vi "Drive Controller.vi"(8 "error in":errorcluster) -> ()   [LabVIEW 2019]
doc: "This VI executes continuously carrying out the current operation and responding to updates or new operation requests. It will often contain the timing or control code that is difficult to place directly in TeleOp. This VI generally opens all sensors and motors and isolates the rest of the robot code from knowing implementation details of how the operations are carried out."
uses:
  <vilib>/Rock Robotics/WPI/Framework/Completion Status.ctl
  Drive Setpoints.ctl
  Drive Operations.ctl
  <vilib>/Rock Robotics/WPI/SafetyOutput/WPI_SafetyOutputConfigMenu.ctl
  <vilib>/Rock Robotics/SystemInterfaces/DIO/FPGA_DIOChannel.ctl
  <vilib>/Rock Robotics/WPI/Solenoid/WPI_SolenoidChannel.ctl
  <vilib>/Rock Robotics/WPI/Solenoid/WPI_SolenoidValue.ctl
  <vilib>/Rock Robotics/WPI/Counter/WPI_CounterDigitalInputToDigitalSource.vi
  <vilib>/Rock Robotics/WPI/Solenoid/WPI_SolenoidOpenDouble.vi
  <vilib>/Rock Robotics/WPI/Solenoid/WPI_SolenoidSetEnum.vi
  <vilib>/Rock Robotics/WPI/RobotDrive/WPI_RobotDriveOpen4MotorWithExistingMotors.vi
  Drive Globals.vi
  <vilib>/Rock Robotics/WPI/RobotDrive/WPI_RobotDriveOpen2MotorWithVictorSPX.vi
panel:
  out "Right Drive Velocity":dbl
  out "Left Drive Velocity":dbl
  in  "Interactive Values":T1
  in  "Buttons":cluster{"Execute Cmd":bool, "Abort Cmd":bool}
  out "Command Timing":cluster{"Start Time (ms)":u32, "Iterations":i32}
  out "Status":T3
  out "Setpoints":T4(graph)
  out "Current\nCmd":string
  # "Tip: The graph shows the motor setpoints. It may also be helpful to observe inputs and sensor values.\nYou may also want to display tuning or debugging controls."
  # "Interactive Command: You may fill in the settings for a command\nand schedule it with the Execute button. You can observe and abort\nany command while fine tuning the code for the controller."
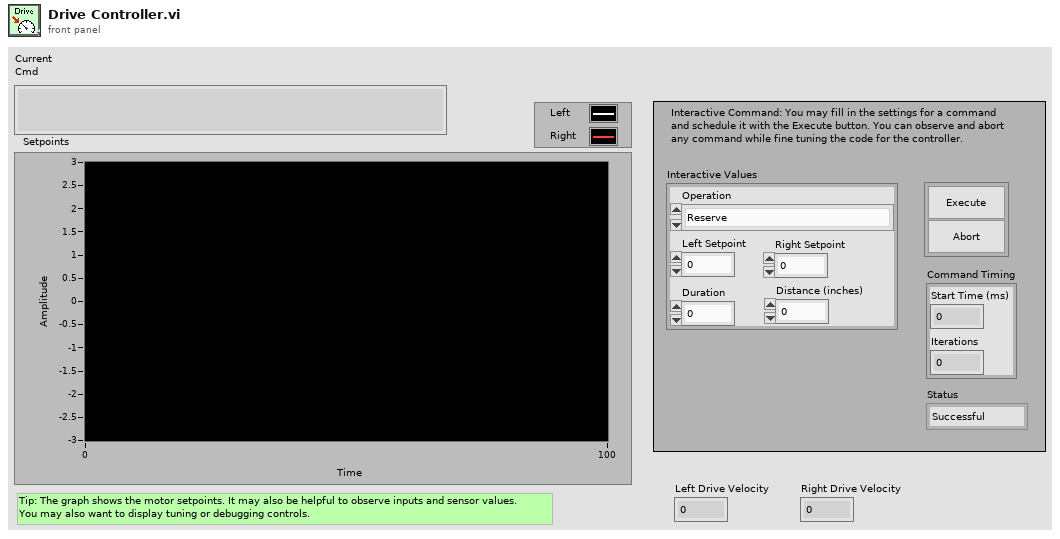
[diagram p1: front panel]
types:
  T1 = typedef "Drive Setpoints.ctl" = cluster{"Operation":T2, "Left Setpoint":dbl, "Right Setpoint":dbl, "Duration":dbl, "Distance (inches)":dbl}
  T2 = typedef "Drive Operations.ctl" = enum16{"Reserve", "Read Current", "Immediate", "Drive for Time", "Drive for Distance"}
  T3 = typedef "Completion Status.ctl" = enum16{"Successful", "Aborted", "Incomplete"}
  T4 = cluster{"Left Setpoint":dbl, "Right Setpoint":dbl}
  T5 = typedef "WPI_SolenoidValue.ctl" = enum16{"Off", "On", "Forward", "Reverse"}
  T6 = typedef "WPI_SolenoidChannel.ctl" = enum8{"Solenoid 0", "Solenoid 1", "Solenoid 2", "Solenoid 3", "Solenoid 4", "Solenoid 5", "Solenoid 6", "Solenoid 7", "Invalid"}
  T7 = typedef "FPGA_DIOChannel.ctl" = enum8{"DIO 0", "DIO 1", "DIO 2", "DIO 3", "DIO 4", "DIO 5", "DIO 6", "DIO 7", "DIO 8", "DIO 9", "DIO MXP 0", "DIO MXP 1", "DIO MXP 2", "DIO MXP 3", "DIO MXP 4", "DIO MXP 5", "DIO MXP 6", "DIO MXP 7", "DIO MXP 8", "DIO MXP 9", "DIO MXP 10", "DIO MXP 11", "DIO MXP 12", "DIO MXP 13", "DIO MXP 14", "DIO MXP 15", "SPI Port CS1", "SPI Port CS2", "SPI Port CS3", "SPI Port MISO", "SPI Port MOSI", "Invalid"}
  T8 = typedef "WPI_SafetyOutputConfigMenu.ctl" = enum16{"Enable", "Disable"}
  T9 = typedef "WPI_MotorControlDeviceRef.ctl" = cluster{"DeviceStatus":errorcluster, "Type":T10, "PWM":cluster{"PWM Channel":T11, "DeadBand":T12}, "CAN":cluster{"Device Number":u8, "SetOutput VI Ref":variant, "GetOutput VI Ref":variant, "Enable VI Ref":variant, "Disable VI Ref":variant, "Data":variant}, "Invert":bool, "DIO PWM":cluster{"PWM \"Enable\" Channel":T11, "DIOChannel":T7, "PWM Rate":dbl}}
  T10 = typedef "WPI_MotorControlType.ctl" = enum16{"PWM", "CAN", "DIO PWM"}
  T11 = typedef "FPGA_DIOPWMChannel.ctl" = enum8{"PWM 0", "PWM 1", "PWM 2", "PWM 3", "PWM 4", "PWM 5", "PWM 6", "PWM 7", "PWM 8", "PWM 9", "PWM MXP 0", "PWM MXP 1", "PWM MXP 2", "PWM MXP 3", "PWM MXP 4", "PWM MXP 5", "PWM MXP 6", "PWM MXP 7", "PWM MXP 8", "PWM MXP 9", "Invalid"}
  T12 = typedef "WPI_PWMDeadband.ctl" = cluster{"Name":string, "maxPositivePwm":i32, "minPositivePwm":i32, "centerPwm":i32, "maxNegativePwm":i32, "minNegativePwm":i32, "angularRange":u16}
  T13 = typedef "WPI_DigitalInputDevRef.ctl" = cluster{"DevStatus":errorcluster, "DIO Channel":T7}
  T14 = typedef "FPGA_CounterEncoderSourceConvertionLVSourceType.ctl" = cluster{"DevStatus":errorcluster, "AnalogTriggerMode?":bool, "DigitalMode":cluster{"DIO Channel":T15}, "AnalogTriggerMode":cluster{"AnalogTriggerIndex":T16, "OutputType":T17}}
  T15 = typedef "FPGA_DIODigitalSourceChannel.ctl" = enum8{"DIO 0", "DIO 1", "DIO 2", "DIO 3", "DIO 4", "DIO 5", "DIO 6", "DIO 7", "DIO 8", "DIO 9", "DIO MXP 0", "DIO MXP 1", "DIO MXP 2", "DIO MXP 3", "DIO MXP 4", "DIO MXP 5", "DIO MXP 6", "DIO MXP 7", "DIO MXP 8", "DIO MXP 9", "DIO MXP 10", "DIO MXP 11", "DIO MXP 12", "DIO MXP 13", "DIO MXP 14", "DIO MXP 15", "SPI Port CS1", "SPI Port CS2", "SPI Port CS3", "SPI Port MISO", "SPI Port MOSI", "Disabled"}
  T16 = typedef "FPGA_AnalogTriggerIndex.ctl" = enum8{"Trig 0", "Trig 1", "Trig 2", "Trig 3", "Trig 4", "Trig 5", "Trig 6", "Trig 7", "Invalid"}
  T17 = typedef "FPGA_AnalogTriggerOutType.ctl" = enum16{"InWindow", "TriggerState", "Rising", "Falling"}
  T18 = typedef "WPI_RobotDriveDevRef.ctl" = cluster{"DevStatus":errorcluster, "Motors[]":T9[], "Square Inputs":bool, "Max Output":dbl}
  T19 = typedef "WPI_SolenoidDevRef.ctl" = cluster{"DevStatus":errorcluster, "Pneumatics Control Module":u8, "Forward Solenoid Channel":T6, "Reverse Solenoid Channel":T6}
  T20 = typedef "WPI_EncoderDevRef.ctl" = cluster{"DevStatus":errorcluster, "EncoderIndex":T21, "CounterIndex":T22, "DistancePerCount":dbl, "Decoding Type":T23}
  T21 = typedef "FPGA_EncoderIdx.ctl" = enum8{"Enc 0", "Enc 1", "Enc 2", "Enc 3", "Enc 4", "Enc 5", "Enc 6", "Enc 7", "Invalid"}
  T22 = typedef "FPGA_CounterCtrSystemIndex.ctl" = enum8{"Ctr 0", "Ctr 1", "Ctr 2", "Ctr 3", "Ctr 4", "Ctr 5", "Ctr 6", "Ctr 7", "Invalid"}
  T23 = typedef "WPI_EncoderType.ctl" = enum16{"1x", "2x", "4x"}
  T24 = typedef "Command Status Info.ctl" = cluster{"Name":string, "Status":T3, "notifier out":T25}
  T25 = typedef "Completion Notifier.ctl" = refnum<notifier>
  T26 = cluster{"SubSystem Data":T1, cluster{"Start Time (ms)":u32, "Iterations":i32}, cluster{"Command Info":T24, "Description":string, "Default Command":T1, "queue out":refnum<queue>, "Subsystem Name":string}}
  T27 = cluster{"SubSystem Data":T1, cluster{"Start Time (ms)":u32, "Iterations":i32}, "Default Command Arguments":cluster{"Command Info":T24, "Description":string, "Default Command":T1, "queue out":refnum<queue>, "Subsystem Name":string}}
  T28 = cluster{"Sensor Velocity":dbl, "Sensor Velocity":dbl}
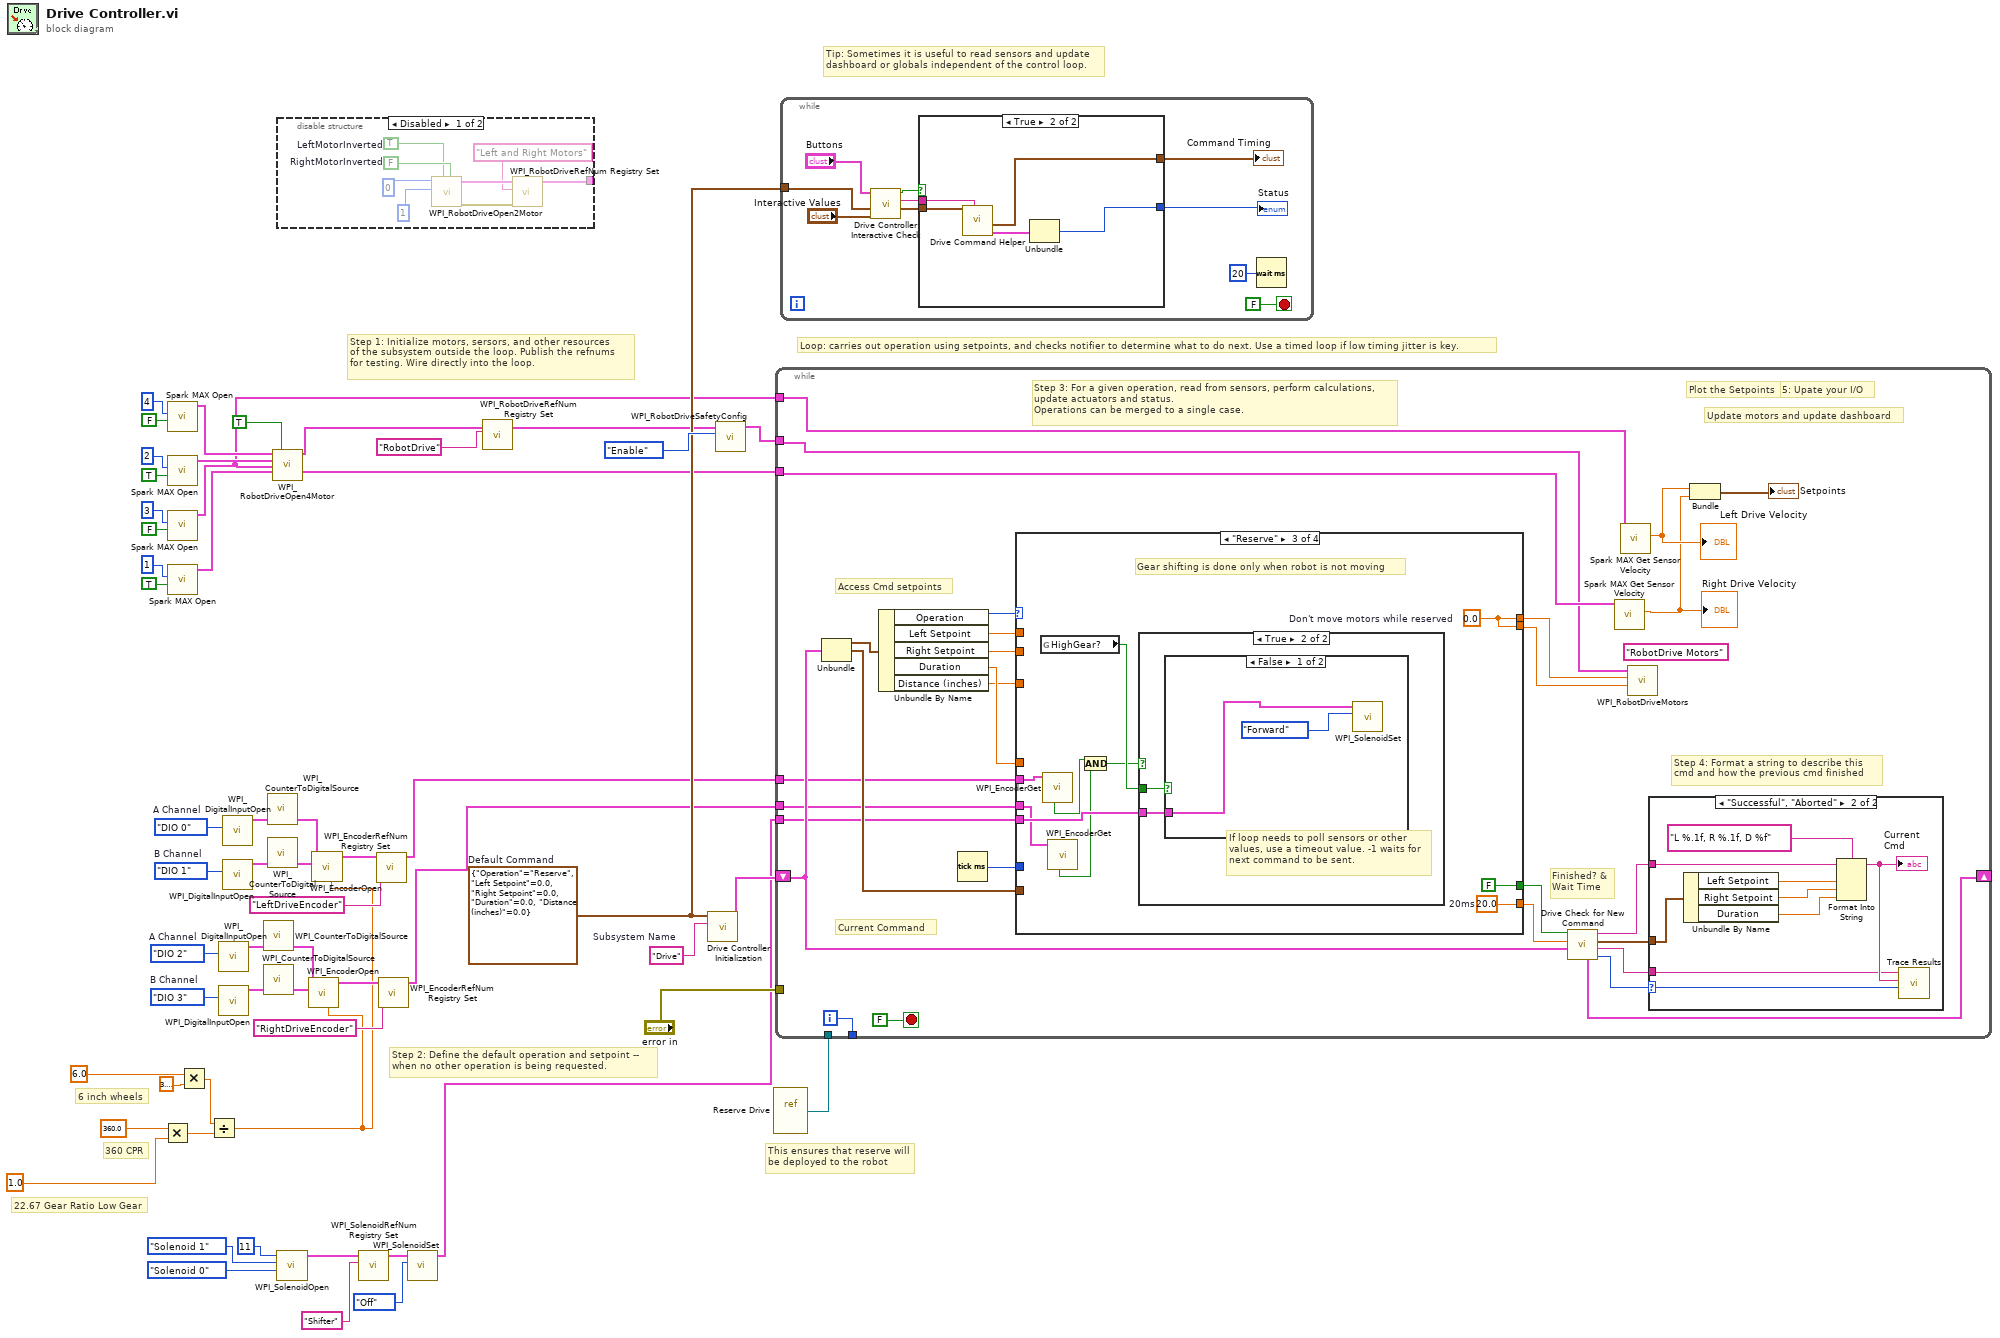
[diagram p0: block diagram]
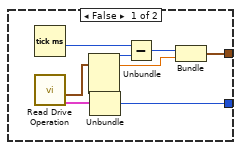
[diagram p3: hidden frame]
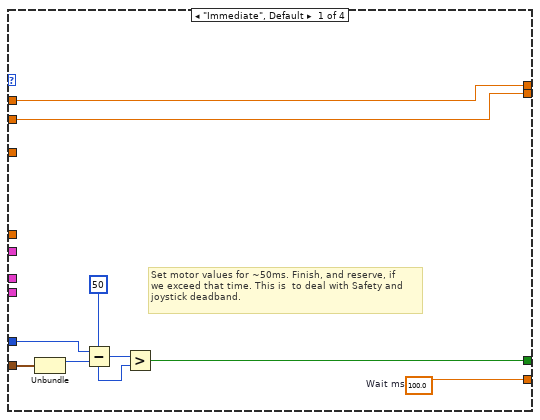
[diagram p5: hidden frame]
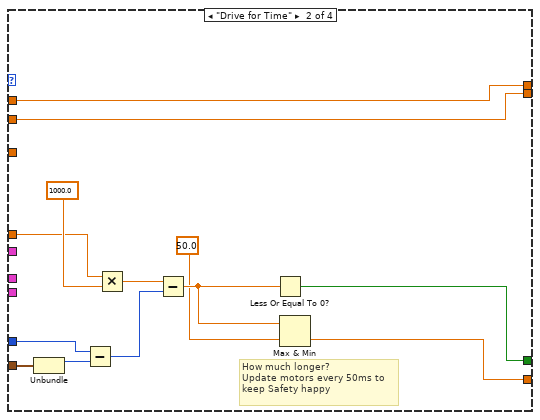
[diagram p6: hidden frame]
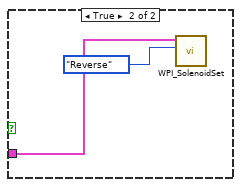
[diagram p8: hidden frame]
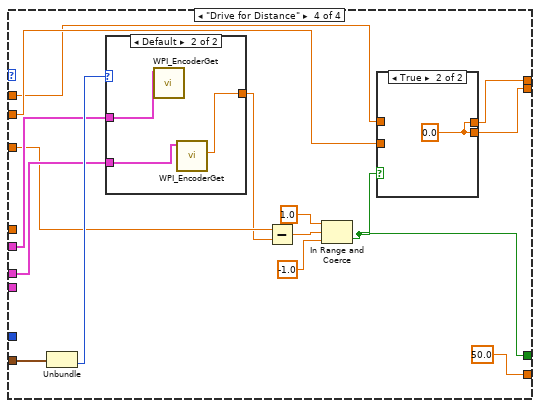
[diagram p9: hidden frame]
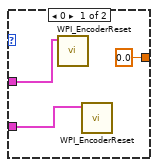
[diagram p11: hidden frame]
diagram:
  w33 = FPGA_DIOChannel."DIO 3"  # B Channel
  w32 = FPGA_DIOChannel."DIO 2"  # A Channel
  w39 = FPGA_DIOChannel."DIO 1"  # B Channel
  w38 = FPGA_DIOChannel."DIO 0"  # A Channel
  w50 = T1 {"Operation"=enum."Reserve", "Left Setpoint"=0.0, "Right Setpoint"=0.0, "Duration"=0.0, "Distance (inches)"=0.0}  # Default Command
  w56 = "Drive"  # Subsystem Name
  # "6 inch wheels"
  # "22.67 Gear Ratio Low Gear"
  # "360 CPR"
  # "This ensures that reserve will\nbe deployed to the robot"
  # "Tip: Sometimes it is useful to read sensors and update\ndashboard or globals independent of the control loop."
  # "Step 2: Define the default operation and setpoint --\nwhen no other operation is being requested."
  # "Step 1: Initialize motors, sersors, and other resources\nof the subsystem outside the loop. Publish the refnums\nfor testing. Wire directly into the loop."
  # "Loop: carries out operation using setpoints, and checks notifier to determine what to do next. Use a timed loop if low timing jitter is key."
  n1 = Multiply(x=360.0, y=1.0) -> (x*y=w4:dbl)
  n2 = call <vilib>:"Spark MAX Open.vi"("Invert"=FALSE, "Device Number"=u8 4) -> ("MotorControlDeviceRef"=w40:T9)  [unwired: 8 in, 1 out]
  n3 = call <vilib>:"Spark MAX Open.vi"("Invert"=TRUE, "Device Number"=u8 2) -> ("MotorControlDeviceRef"=w41:T9)  [unwired: 8 in, 1 out]
  n4 = call <vilib>:"Spark MAX Open.vi"("Invert"=FALSE, "Device Number"=u8 3) -> ("MotorControlDeviceRef"=w2:T9)  [unwired: 8 in, 1 out]
  n5 = call <vilib>:"Spark MAX Open.vi"("Invert"=TRUE, "Device Number"=u8 1) -> ("MotorControlDeviceRef"=w1:T9)  [unwired: 8 in, 1 out]
  n6 = Multiply(x=6.0 ("DistancePerCount"), y=3.141592653589793) -> (x*y=w5:dbl)
  n7 = Divide(x=w5, y=w4) -> (x/y=w3:dbl)
  n8 = call <vilib>:"WPI_DigitalInputOpen.vi"("DIO Channel"=w32) -> ("DigitalInputDevRef"=w29:T13)  [unwired: 1 in, 9 out]
  n9 = call <vilib>:"WPI_DigitalInputOpen.vi"("DIO Channel"=w33) -> ("DigitalInputDevRef"=w30:T13)  [unwired: 1 in, 9 out]
  n10 = call <vilib>:"WPI_DigitalInputOpen.vi"("DIO Channel"=w38) -> ("DigitalInputDevRef"=w35:T13)  [unwired: 1 in, 9 out]
  n11 = call <vilib>:"WPI_DigitalInputOpen.vi"("DIO Channel"=w39) -> ("DigitalInputDevRef"=w36:T13)  [unwired: 1 in, 9 out]
  n12 = call-poly <vilib>:"WPI_CounterToDigitalSource.vi"("DigitalInputDevRef"=w29) -> ("Digital Source"=w28:T14)  [unwired: 6 out]
  n13 = call-poly <vilib>:"WPI_CounterToDigitalSource.vi"("DigitalInputDevRef"=w30) -> ("Digital Source"=w31:T14)  [unwired: 6 out]
  n14 = call-poly <vilib>:"WPI_CounterToDigitalSource.vi"("DigitalInputDevRef"=w35) -> ("Digital Source"=w34:T14)  [unwired: 6 out]
  n15 = call-poly <vilib>:"WPI_CounterToDigitalSource.vi"("DigitalInputDevRef"=w36) -> ("Digital Source"=w37:T14)  [unwired: 6 out]
  n16 = call-poly <vilib>:"WPI_RobotDriveOpen4Motor.vi"("Rear Left Motor Dev Ref"=w40, "Square Inputs"=TRUE, "Rear Right Motor Dev Ref"=w41, "Front Left Motor Dev Ref"=w2, "Front Right Motor Dev Ref"=w1) -> ("RobotDriveDevRef"=w43:T18)  [unwired: 9 in, 1 out]
  n17 = call-poly <vilib>:"WPI_SolenoidOpen.vi"("Reverse Solenoid Channel"=WPI_SolenoidChannel."Solenoid 0", "Forward Solenoid Channel"=WPI_SolenoidChannel."Solenoid 1", "Pneumatics Control Module (0)"=11) -> ("SolenoidDevRef"=w19:T19)  [unwired: 7 in, 1 out]
  n18 = disable-structure shown="Disabled" {
    disable-tunnel: [w57 _] -> _
    frame Disabled {
      w61 = TRUE  # LeftMotorInverted
      w62 = FALSE  # RightMotorInverted
      n19 = call-poly <vilib>:"WPI_RobotDriveOpen2Motor.vi"("Right Motor Inverted"=w62, "Left Motor Inverted"=w61, "Right Motor"=u8 1 ("Left Motor"), "Left Motor"=u8 0) -> ("error out"=w58:errorcluster, "RobotDriveDevRef"=w60:T18)  [unwired: 1 in, 5 out]
      n20 = call <vilib>:"WPI_RobotDriveRefNum Registry Set.vi"("error in (no error)"=w58, "refnum name"="Left and Right Motors", "RobotDriveDevRef"=w60) -> ("RobotDriveDevRef"=w57:T18)  [unwired: 1 in, 7 out]
    }
    frame Enabled {
    }
  }
  n21 = call <vilib>:"WPI_EncoderOpen.vi"("DistancePerCount"=w3, "BSource"=w31, "ASource"=w28) -> ("EncoderDevRef"=w25:T20)  [unwired: 5 in, 3 out]
  n22 = call <vilib>:"WPI_EncoderOpen.vi"("DistancePerCount"=w3, "BSource"=w37, "ASource"=w34) -> ("EncoderDevRef"=w27:T20)  [unwired: 5 in, 3 out]
  n23 = call <vilib>:"WPI_SolenoidRefNum Registry Set.vi"("refnum name"="Shifter", "SolenoidDevRef"=w19) -> ("SolenoidDevRef"=w18:T19)  [unwired: 8 in, 1 out]
  n24 = call <vilib>:"WPI_EncoderRefNum Registry Set.vi"("refnum name"="LeftDriveEncoder", "EncoderDevRef"=w27) -> ("EncoderDevRef"=w23:T20)  [unwired: 8 in, 1 out]
  n25 = call <vilib>:"WPI_EncoderRefNum Registry Set.vi"("refnum name"="RightDriveEncoder", "EncoderDevRef"=w25) -> ("EncoderDevRef"=w14:T20)  [unwired: 8 in, 1 out]
  n26 = call-poly <vilib>:"WPI_SolenoidSet.vi"("Value"=WPI_SolenoidValue."Off", "SolenoidDevRef"=w18) -> ("SolenoidDevRef"=w15:T19)  [unwired: 8 in, 1 out]
  n27 = call <vilib>:"WPI_RobotDriveRefNum Registry Set.vi"("refnum name"="RobotDrive", "RobotDriveDevRef"=w43) -> ("RobotDriveDevRef"=w44:T18)  [unwired: 2 in, 7 out]
  n28 = call "Drive Controller Initialization.vi"("Subsystem Name"=w56, "Default Command"=w50) -> ("Current Command"=w52:T26)  [unwired: 9 in]
  n29 = call <vilib>:"WPI_RobotDriveSafetyConfig.vi"("mode"=WPI_SafetyOutputConfigMenu."Enable", "RobotDriveDevRef"=w44) -> ("RobotDriveDevRef"=w54:T18)  [unwired: 8 in, 1 out]
  n30 = vi-ref "Reserve Drive.vi"() -> (w51:refnum<vi>)
  n31 = while {
    shift-right: [w81] -> _
    shift-left: w52 -> [w74]
    tunnel: [w92] -> _
    tunnel: w54 -> [w66]
    tunnel: "error in" -> [_]
    tunnel: w51 -> [_]
    tunnel: w23 -> [w73]
    tunnel: w15 -> [w72]
    tunnel: w14 -> [w71]
    tunnel: w2 -> [w69]
    tunnel: w1 -> [w68]
    i -> [w92]
    stop <- FALSE stop-if-true
    (unwired) "RobotDrive Motors" ("Name")
    # "Step 5: Upate your I/O"
    # "Step 4: Format a string to describe this\ncmd and how the previous cmd finished"
    # "Current Command"
    # "Update motors and update dashboard"
    # "Plot the Setpoints"
    # "Access Cmd setpoints"
    # "Finished? &\nWait Time"
    # "Step 3: For a given operation, read from sensors, perform calculations,\nupdate actuators and status.\nOperations can be merged to a single case."
    n32 = Unbundle(w74) -> ("SubSystem Data"=w88:T1, w75:cluster{"Start Time (ms)":u32, "Iterations":i32})  [unwired: 1 out]
    n33 = Unbundle By Name(w88) -> ("Operation"=w87:T2, "Left Setpoint"=w86:dbl, "Right Setpoint"=w85:dbl, "Duration"=w84:dbl, "Distance (inches)"=w70:dbl)
    n34 = Tick Count (ms)() -> (millisecond timer value=w83:u32)
    n35 = case shown="\"Reserve\"" w87 {
      tunnel: [w111 w112 w134 50.0 ("20ms")] -> w80
      tunnel: [w104 w119 FALSE ("ignore previous (F)") w144] -> w79
      tunnel: w75 -> [w103 w121 _ w155]
      tunnel: [w110 w118 w132 w148] -> w90
      tunnel: [w109 w117 w132 w149] -> w89
      tunnel: w86 -> [w110 w118 _ w150]
      tunnel: w85 -> [w109 w117 _ w151]
      tunnel: w84 -> [_ w116 _ _]
      tunnel: w83 -> [w105 w115 _ _]
      tunnel: w73 -> [_ _ w131 w153]
      tunnel: w72 -> [_ _ w130 _]
      tunnel: w71 -> [_ _ w127 w152]
      tunnel: w70 -> [_ _ _ w146]
      frame "Immediate", Default {
        w111 = 100.0  # Wait ms
        # "Set motor values for ~50ms. Finish, and reserve, if\nwe exceed that time. This is  to deal with Safety and\njoystick deadband."
        n36 = Unbundle(w103) -> ("Start Time (ms)"=w106:u32)  [unwired: 1 out]
        n37 = Subtract(x=w105, y=w106) -> (x-y=w107:u32)
        n38 = Greater?(x=w107, y=u8 50 ("Left Motor")) -> (0:w104:bool)
      }
      frame "Drive for Time" {
        # "How much longer?\nUpdate motors every 50ms to\nkeep Safety happy"
        n39 = Unbundle(w121) -> ("Start Time (ms)"=w120:u32)  [unwired: 1 out]
        n40 = Subtract(x=w115, y=w120) -> (x-y=w124:u32)
        n41 = Multiply(x=w116, y=1000.0) -> (x*y=w123:dbl)
        n42 = Subtract(x=w123, y=w124) -> (x-y=w114:dbl)
        n43 = Less Or Equal To 0?(x=w114) -> (x <= 0?=w119:bool)
        n44 = Max & Min(x=w114, y=50.0) -> (min(x,y)=w112:dbl)  [unwired: 1 out]
      }
      frame "Reserve" {
        w132 = 0.0  # Don't move motors while reserved
        w134 = 20.0  # 20ms
        # "Gear shifting is done only when robot is not moving"
        n45 = global read "Drive Globals.vi" "HighGear?"() -> (w129:bool)
        n46 = call <vilib>:"WPI_EncoderGet.vi"("EncoderDevRef"=w131) -> ("Stopped"=w128:bool)  [unwired: 5 in, 5 out]
        n47 = call <vilib>:"WPI_EncoderGet.vi"("EncoderDevRef"=w127) -> ("Stopped"=w126:bool)  [unwired: 5 in, 5 out]
        n48 = And(x=w128, y=w126) -> (x .and. y?=w125:bool)
        n49 = case shown="True" w125 {
          tunnel: w130 -> [_ w136]
          tunnel: w129 -> [_ w135]
          frame False {
          }
          frame True {
            # "If loop needs to poll sensors or other\nvalues, use a timeout value. -1 waits for\nnext command to be sent."
            n50 = case shown="False" w135 {
              tunnel: w136 -> [w137 w140]
              frame False {
                n51 = call-poly <vilib>:"WPI_SolenoidSet.vi"("Value"=WPI_SolenoidValue."Forward", "SolenoidDevRef"=w137) -> ()  [unwired: 8 in, 2 out]
              }
              frame True {
                n52 = call-poly <vilib>:"WPI_SolenoidSet.vi"("Value"=WPI_SolenoidValue."Reverse", "SolenoidDevRef"=w140) -> ()  [unwired: 8 in, 2 out]
              }
            }
          }
        }
      }
      frame "Drive for Distance" {
        n53 = Unbundle(w155) -> ("Iterations"=w154:i32)  [unwired: 1 out]
        n54 = case shown="Default" w154 {
          tunnel: w153 -> [w161 w164]
          tunnel: w152 -> [w160 w163]
          tunnel: [0.0 ("Distance") w162] -> w145
          frame 0 {
            n55 = call <vilib>:"WPI_EncoderReset.vi"("EncoderDevRef"=w161) -> ()  [unwired: 9 in, 2 out]
            n56 = call <vilib>:"WPI_EncoderReset.vi"("EncoderDevRef"=w160) -> ()  [unwired: 9 in, 2 out]
          }
          frame Default {
            n57 = call <vilib>:"WPI_EncoderGet.vi"("EncoderDevRef"=w164) -> ()  [unwired: 5 in, 6 out]
            n58 = call <vilib>:"WPI_EncoderGet.vi"("EncoderDevRef"=w163) -> ("Distance"=w162:dbl)  [unwired: 5 in, 5 out]
          }
        }
        n59 = Subtract(x=w146, y=w145) -> (x-y=w143:dbl)
        n60 = In Range and Coerce(upper limit=1.0, x=w143, lower limit=-1.0) -> (In Range?=w144:bool)  [unwired: 1 out]
        n61 = case shown="True" w144 {
          tunnel: w151 -> [w156 _]
          tunnel: w150 -> [w157 _]
          tunnel: [w156 w158] -> w149
          tunnel: [w157 w158] -> w148
          frame False {
          }
          frame True {
            w158 = 0.0
          }
        }
      }
    }
    n62 = call "Drive Check for New Command.vi"("input cluster"=w74, "Wait time (ms)"=w80, "Finished?"=w79) -> ("Completion"=w82:T3, "Subsystem Name"=w76:string, "Current Command"=w77:T1, "Initial Trace String"=w78:string, "Next Command"=w81:T27)  [unwired: 4 in]
    n63 = call <vilib>:"Spark MAX Get Sensor Velocity.vi"("MotorControlDevRef in"=w68) -> ("Sensor Velocity"=w65:dbl)  [unwired: 7 in, 3 out]
    "Right Drive Velocity" <- w65
    n64 = call <vilib>:"Spark MAX Get Sensor Velocity.vi"("MotorControlDevRef in"=w69) -> ("Sensor Velocity"=w67:dbl)  [unwired: 7 in, 3 out]
    "Left Drive Velocity" <- w67
    n65 = call <vilib>:"WPI_RobotDriveMotors.vi"("RightSpeed"=w89, "LeftSpeed"=w90, "RobotDriveDevRef"=w66) -> ()  [unwired: 1 in, 8 out]
    n66 = case shown="\"Successful\", \"Aborted\"" w82 {
      selector: w82 -> [_ w102]
      tunnel: w78 -> [_ w97]
      tunnel: w77 -> [_ w98]
      tunnel: w76 -> [_ w94]
      frame "Incomplete", Default {
        # "Continuing current command"
      }
      frame "Successful", "Aborted" {
        # "Report and setup for next command"
        n67 = Unbundle By Name(w98) -> ("Left Setpoint"=w100:dbl, "Right Setpoint"=w101:dbl, "Duration"=w95:dbl)
        n68 = Format Into String(format string="L %.1f, R %.1f, D %f", initial string=w97, w100, w101, w95) -> (resulting string=w96:string)  [unwired: 1 in, 1 out]
        "Current\nCmd" <- w96
        n69 = call <vilib>:"Trace Results.vi"("Status of previous command"=w102, "Description"=w96, "Subsystem"=w94) -> ()  [unwired: 9 in]
      }
    }
    n70 = Bundle("Sensor Velocity"=w67, "Sensor Velocity"=w65) -> (→"Setpoints":T28)  [unwired: 1 in]
  }
  n71 = while {
    tunnel: w50 -> [w166]
    stop <- FALSE stop-if-true
    n72 = call "Drive Controller Interactive Check.vi"("Interactive Command In"="Interactive Values", "Default Command"=w166, "Buttons"="Buttons") -> ("Interactive Command Out"=w168:T1, "Trace String"=w169:string, "Schedule"=w170:bool)  [unwired: 6 in]
    n73 = case shown="True" w170 {
      tunnel: [w179 w187] -> w171
      tunnel: [w178 w183] -> w172
      tunnel: w169 -> [_ w185]
      tunnel: w168 -> [_ w184]
      frame False {
        n74 = Tick Count (ms)() -> (millisecond timer value=w182:u32)
        n75 = call "Read Drive Operation.vi"() -> ("Command Info"=w176:T24, "SubSystem Data"=w175:T1)  [unwired: 9 in, 1 out]
        n76 = Unbundle(w175) -> ("Operation"=w180:T2, "Left Setpoint"=w177:dbl)  [unwired: 3 out]
        n77 = Unbundle(w176) -> ("Status"=w179:T3)  [unwired: 2 out]
        n78 = Subtract(x=w182, y=w180) -> (x-y=w181:u32)
        n79 = Bundle(w181, "Left Setpoint"=w177) -> (w178:cluster{u32, "Left Setpoint":dbl})  [unwired: 1 in]
      }
      frame True {
        n80 = call "Drive Command Helper.vi"("Description"=w185, "SubSystem Data"=w184) -> ("Command Info Out"=w186:T24, "Command Timing"=w183:cluster{"Start Time (ms)":u32, "Iterations":i32})  [unwired: 7 in, 1 out]
        n81 = Unbundle(w186) -> ("Status"=w187:T3)  [unwired: 2 out]
      }
    }
    "Status" <- w171
    "Command Timing" <- w172
    n82 = Wait (ms)(milliseconds to wait=u32 20) -> ()  [unwired: 1 out]
  }
